vi "JKI SM EDITOR - quick filter list.vi"(0 "quick filter text":string, 7 "States":string[](array[string]), 11 "error in":errorcluster) -> (6 "All Items Filtered Out":bool, 8 "States quick-filtered":string[](array[string]), 15 "error out":errorcluster)   [LabVIEW 2013]
uses:
  source/source/JKI State Machine API/source/JKI SM/JKI SM.lvclass
panel:
  # "Copyright © 2006 James Kring, Inc. All rights reserved.\nMichael Aivaliotis michael.aivaliotis@jameskring.com\nalternate email: michael@aivaliotis.com\n\nThis library is provided \"AS IS\" , WITHOUT WARRANTIES OR \nCONDITIONS OF ANY KIND, either express or implied.\n\nJames Kring, Inc. -- http://www.jameskring.com"
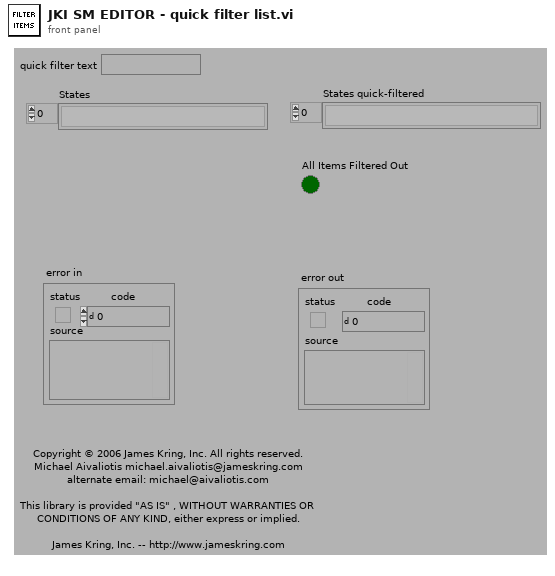
[diagram p1: front panel]
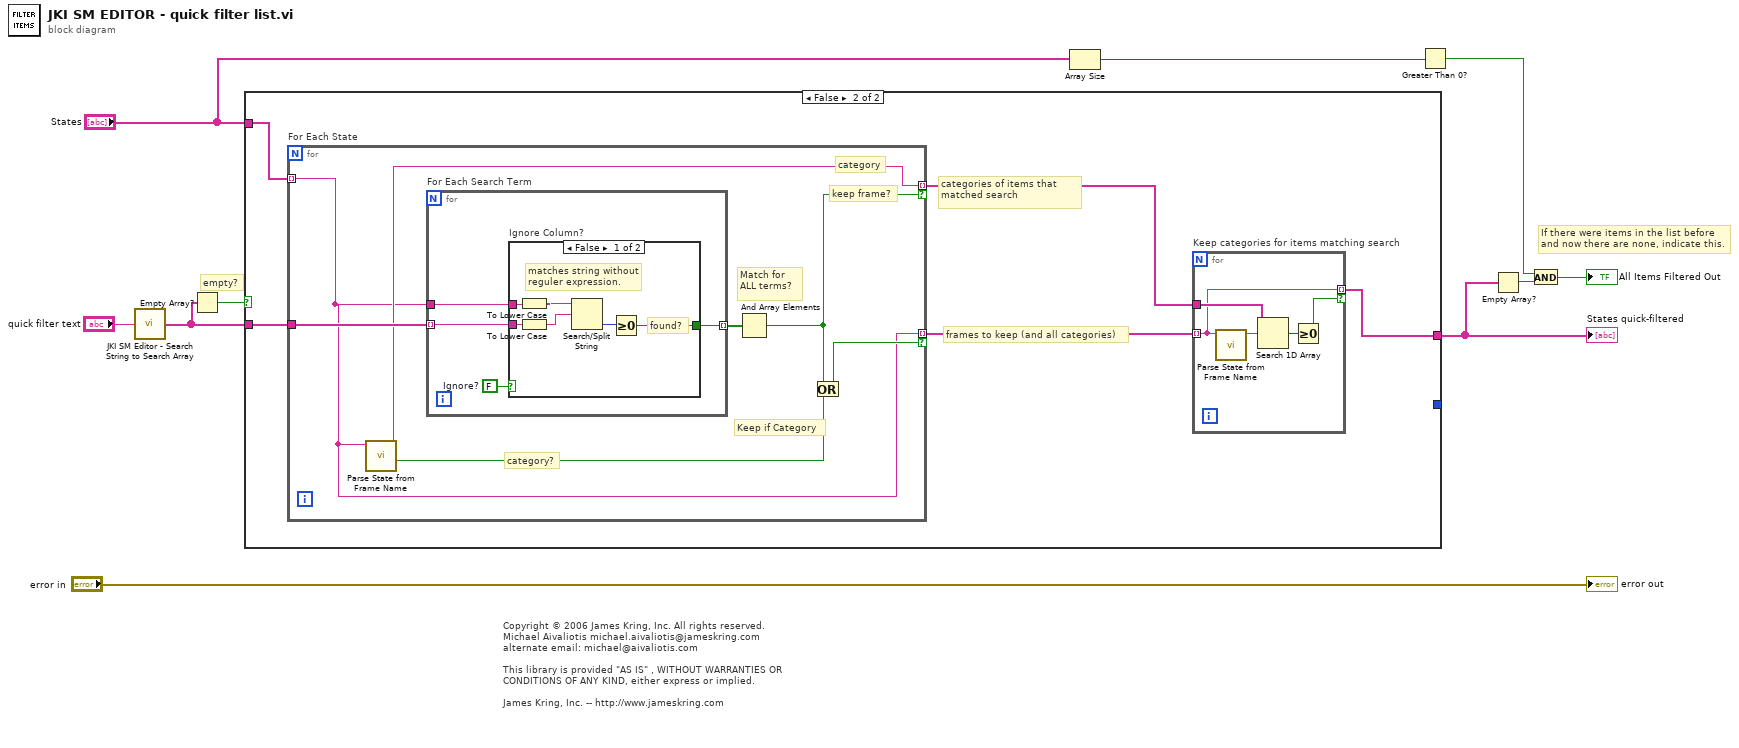
[diagram p0: block diagram]
diagram:
  # "If there were items in the list before and now there are none, indicate this."
  # "Copyright © 2006 James Kring, Inc. All rights reserved.\nMichael Aivaliotis michael.aivaliotis@jameskring.com\nalternate email: michael@aivaliotis.com\n\nThis library is provided \"AS IS\" , WITHOUT WARRANTIES OR \nCONDITIONS OF ANY KIND, either express or implied.\n\nJames Kring, Inc. -- http://www.jameskring.com"
  # "empty?"
  n1 = call "JKI SM Editor - Search String to Search Array.vi"("String"="quick filter text") -> ("Array"=w3:string[])
  n2 = Empty Array?(array=w3) -> (empty?=w2:bool)
  n3 = case shown="False" w2 {
    tunnel: w3 -> [_ w18]
    tunnel: "States" -> [w12 w17]
    tunnel: [w12 w15] -> w9
    tunnel: [w11 _] -> _
    frame True {
      # "return previous list untouched."
      n4 = for {
        tunnel: w12 -> [_] mode=indexing
        tunnel: [w13] -> w11 mode=indexing
        i -> [w13]
      }
    }
    frame False {
      # "categories of items that matched search"
      # "frames to keep (and all categories)"
      n5 = for "For Each State" {
        tunnel: w17 -> [w24] mode=indexing
        tunnel: w18 -> [w30]
        tunnel: [w24] -> w14 mode=indexing if=w27
        tunnel: [w25] -> w16 mode=indexing if=w26
        # "Keep if Category"
        # "category"
        # "keep frame?"
        # "category?"
        # "Match for ALL terms?"
        n6 = call "Parse State from Frame Name.vi"("Frame or State Name"=w24) -> ("is a Category Frame?"=w28:bool, "Category Name"=w25:string)  [unwired: 6 in, 3 out]
        n7 = for "For Each Search Term" {
          tunnel: w24 -> [w34]
          tunnel: w30 -> [w33] mode=indexing
          tunnel: [w32] -> w29 mode=indexing
          w31 = FALSE  # Ignore?
          n8 = case "Ignore Column?" shown="False" w31 {
            tunnel: w34 -> [w40 _]
            tunnel: w33 -> [w39 _]
            tunnel: [w35 _] -> w32
            frame False {
              # "matches string without reguler expression."
              # "found?"
              n9 = To Lower Case(string=w40) -> (all lower case string=w38:string)
              n10 = To Lower Case(string=w39) -> (all lower case string=w37:string)
              n11 = Search/Split String(string=w38, search string/char (-)=w37) -> (offset of match=w36:i32)  [unwired: 1 in, 2 out]
              n12 = Greater Or Equal To 0?(x=w36) -> (x >= 0?=w35:bool)
            }
            frame True {
            }
          }
        }
        n13 = And Array Elements(Boolean array=w29) -> (logical AND=w26:bool)
        n14 = Or(x=w26, y=w28) -> (x .or. y?=w27:bool)
      }
      n15 = for "Keep categories for items matching search" {
        tunnel: w14 -> [w21] mode=indexing
        tunnel: w16 -> [w22]
        tunnel: [w21] -> w15 mode=indexing if=w19
        n16 = call "Parse State from Frame Name.vi"("Frame or State Name"=w21) -> ("Category Name"=w23:string)  [unwired: 6 in, 4 out]
        n17 = Search 1D Array(1D array=w22, element=w23) -> (index of element=w20:i32)  [unwired: 1 in]
        n18 = Greater Or Equal To 0?(x=w20) -> (x >= 0?=w19:bool)
      }
    }
  }
  "States quick-filtered" <- w9
  n19 = Array Size(array="States") -> (size(s)=w5:i32)
  n20 = Greater Than 0?(x=w5) -> (x > 0?=w6:bool)
  n21 = Empty Array?(array=w9) -> (empty?=w8:bool)
  n22 = And(x=w6, y=w8) -> (x .and. y?=→"All Items Filtered Out":bool)
  "error out" <- "error in"
